vi "SPI Master and Slave with debug [FPGA].vi"() -> ()   [LabVIEW 2011]
uses:
  <vilib>/Platform/TimedLoop/XDataNode/timing_clust.ctl
  <vilib>/Platform/TimedLoop/XDataNode/nitl_modes.ctl
  <vilib>/Platform/TimedLoop/XDataNode/wakeup.ctl
  SPI Slave State.ctl
  SPI Master State.ctl
  <vilib>/rvi/interface/RandomDataEmulation/nirviRandomDataFPGAFIFO.vi
  <vilib>/rvi/interface/RandomDataEmulation/niFpgaRandomDataHandleErrors.vi
  <vilib>/Platform/TimedLoop/XDataNode/XDataNode.xnode
  <vilib>/rvi/DataTransferAndStorage/Container/XNode/niFpgaContainer.xnode
  <vilib>/rvi/interface/RandomDataEmulation/nirviRandomDataFpgaReadWriteTemplate.vi
  <vilib>/Platform/TimedLoop/XDataNode/XDNodeRunTimeDep.lvlib
panel:
  out "Slave Data Out":u32
  in  "Slave Data In":u32
  in  "Data Length":u8
  in  "HCP-1":u8
  out "Data Out":u32
  in  "Data In":u32
  in  "TX":bool
  in  "CPOL":bool
  in  "CPHA":bool
  in  "RESET":bool
  out "_SS":bool
  out "SCLK":bool
  out "MOSI":bool
  out "MISO":bool
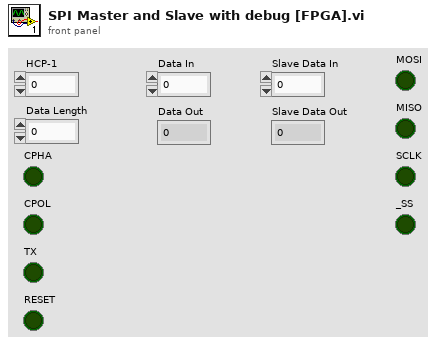
[diagram p1: front panel]
types:
  T1 = typedef "XDNodeRunTimeDep.lvlib/timing_clust.ctl" = cluster{"Expected End [f-1]":u64, "Actual End [f-1]":u64, "Finished Late? [f-1]":bool, "Expected End [i-1]":u64, "Actual End [i-1]":u64, "Finished Late? [i-1]":bool, "Expected Start [i]":u64, "Actual Start [i]":u64, "Expected Start [f]":u64, "Actual Start [f]":u64, "Source Name":string, "Structure Name":string, "Period":i64, "Deadline":i64, "Offset":i64, "Start":i64, "Priority":i32, "Timeout":i32, "Mode":T2, "Wakeup Reason":T3, "Error":errorcluster, "Source Type":string, "Secondary Source Type":string, "Global End Time":u64, "Global Start Time":u64, "Frame Duration":u64, "Iteration Duration":u64, "Assigned CPU":i32, "I/O Scan Engine Mode":u32}
  T2 = typedef "XDNodeRunTimeDep.lvlib/nitl_modes.ctl" = enum32{"No Change", "Process missed periods, maintain original phase", "Discard missed periods, maintain original phase", "Process missed periods, ignore original phase", "Discard missed periods, ignore original phase"}
  T3 = typedef "XDNodeRunTimeDep.lvlib/wakeup.ctl" = enum32{"Normal", "Aborted", "Asynchronous wakeup", "Timing source error", "Timed loop error", "Timeout"}
  T4 = typedef "SPI Slave State.ctl" = enum8{"RESET", "Wait for _SS", "Assert MISO", "Latch MOSI"}
  T5 = typedef "SPI Master State.ctl" = enum8{"RESET", "Wait for TX", "Assert MOSI", "Toggle SCLK", "Latch MISO and Toggle SCLK", "Assert MOSI and Toggle SCLK"}
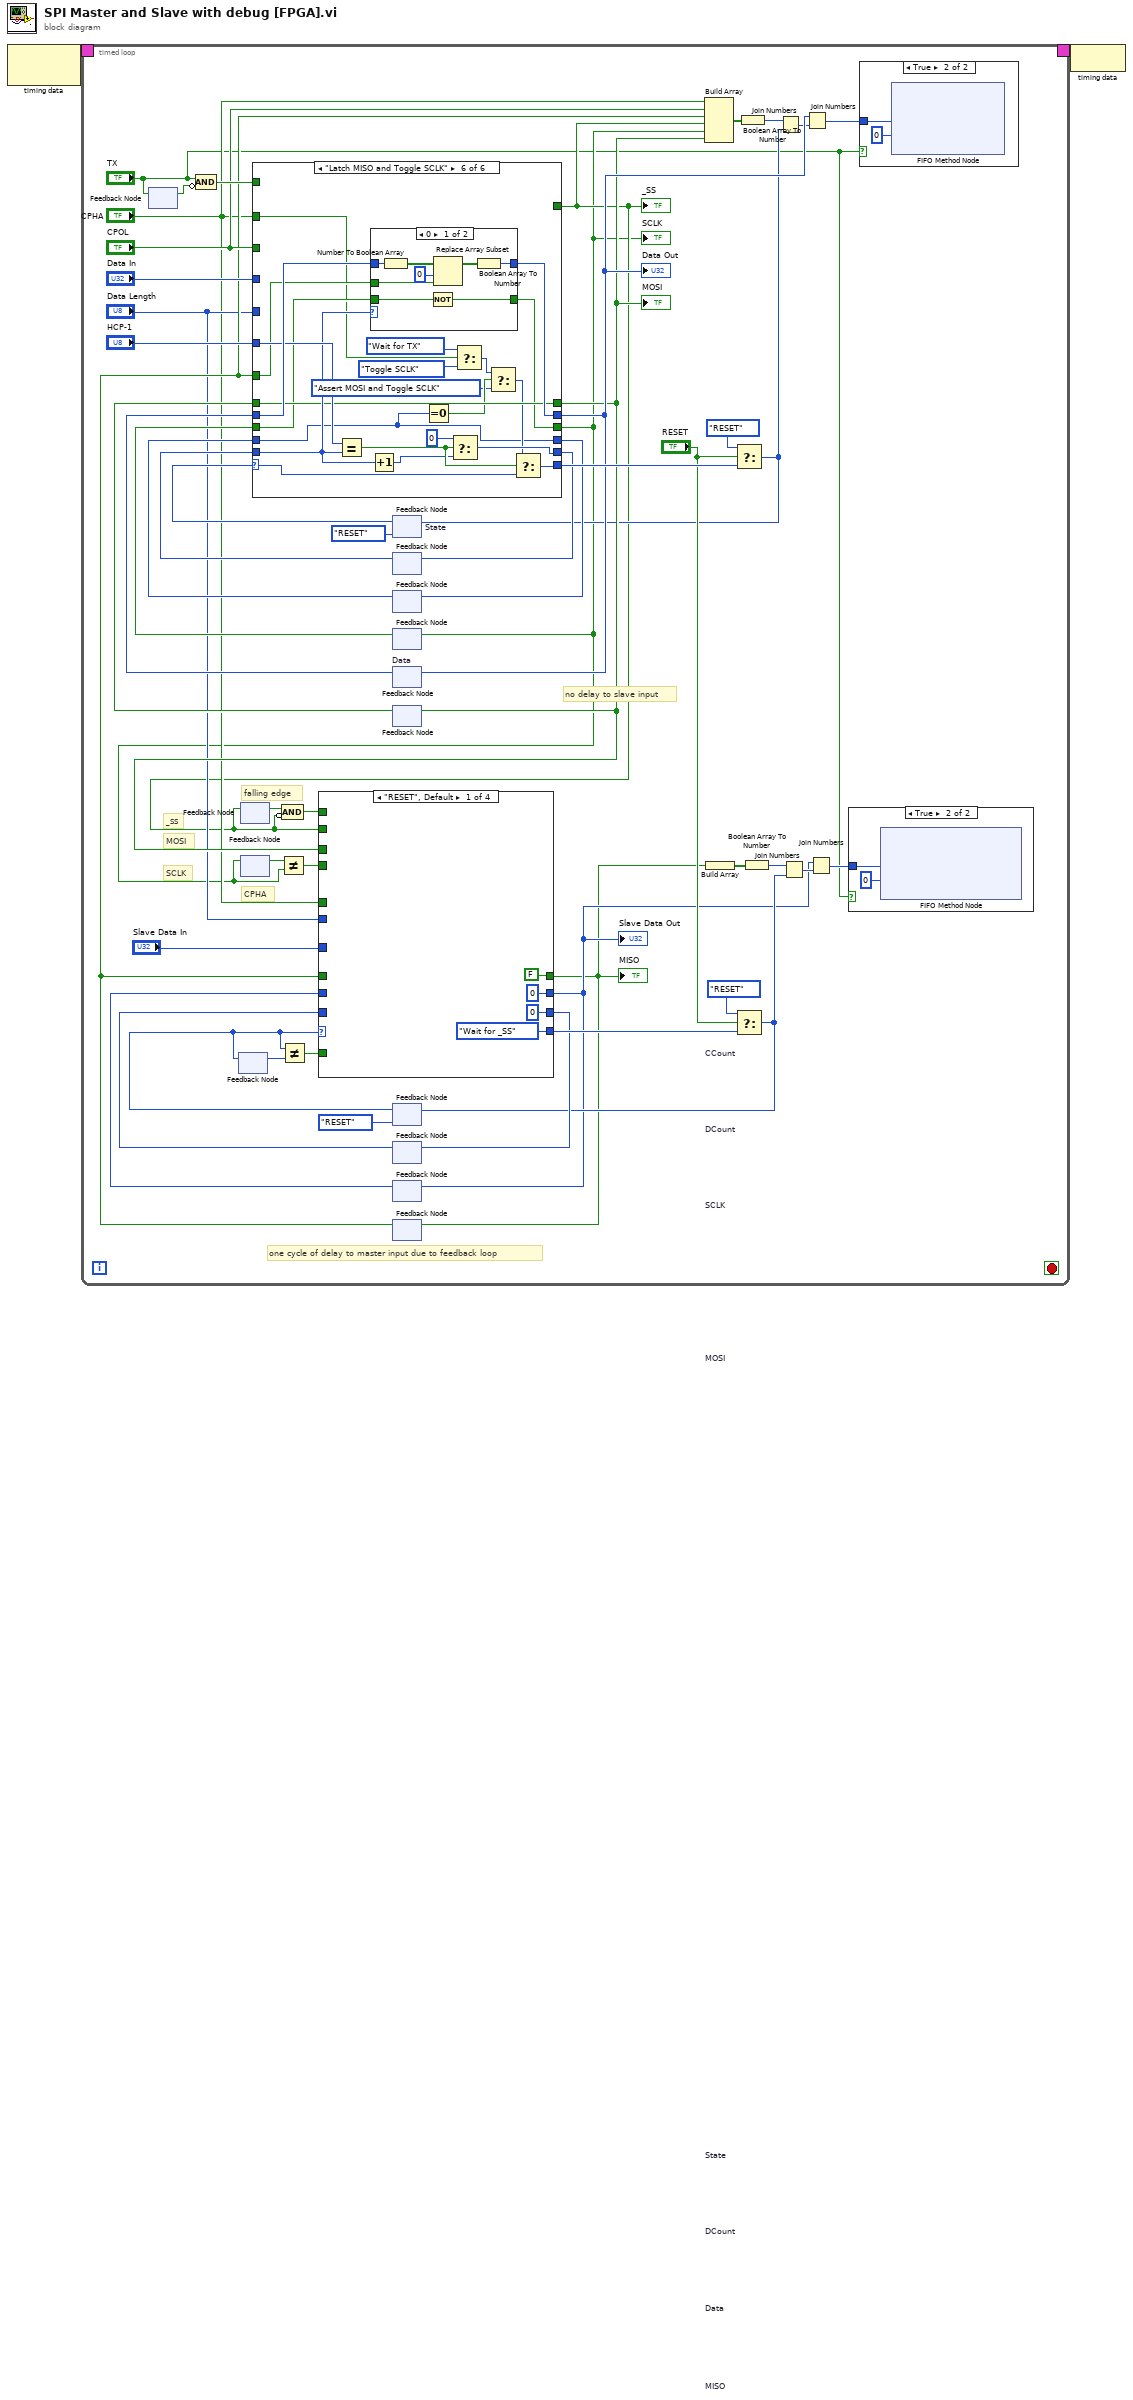
[diagram p0: block diagram]
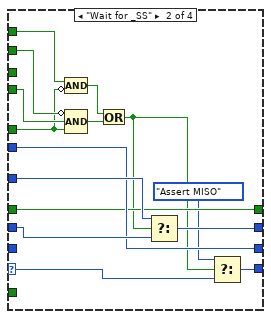
[diagram p3: hidden frame]
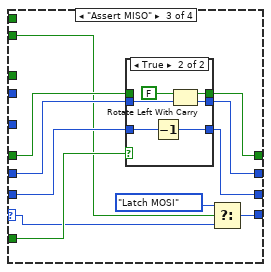
[diagram p4: hidden frame]
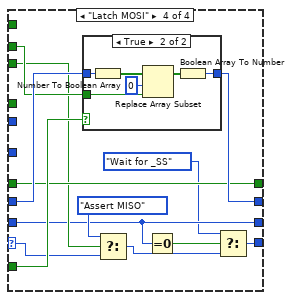
[diagram p6: hidden frame]
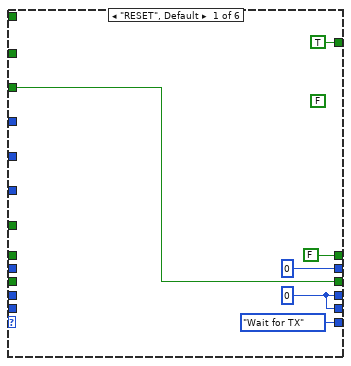
[diagram p9: hidden frame]
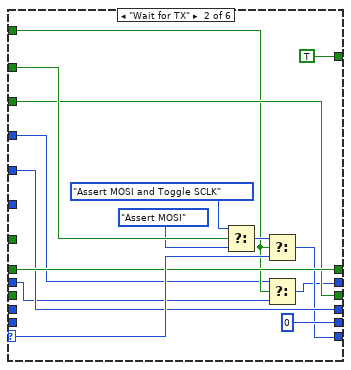
[diagram p10: hidden frame]
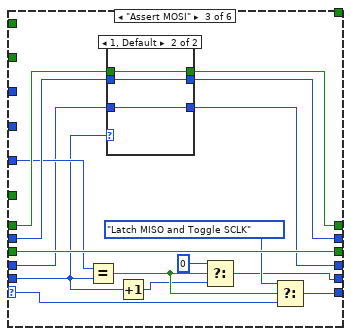
[diagram p11: hidden frame]
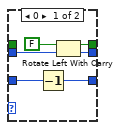
[diagram p12: hidden frame]
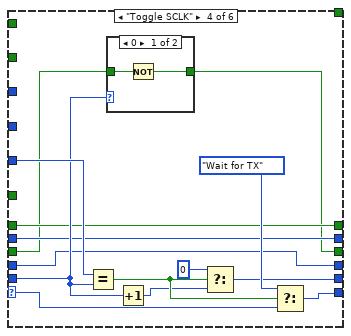
[diagram p13: hidden frame]
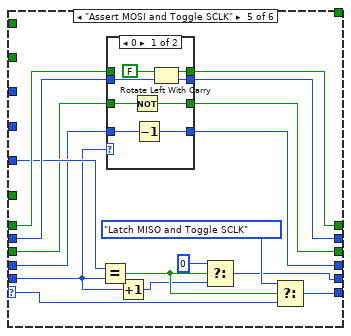
[diagram p15: hidden frame]
diagram:
  n1 = node-c288() -> (w2:T1)  [unwired: 1 in]
  n2 = timed-loop {
    timing: w2 -> [_]
    timing-out: [_] -> w1
    stop <- _ stop-if-true
    # "CPHA"
    # "falling edge"
    # "SCLK"
    # "MOSI"
    # "_SS"
    # "one cycle of delay to master input due to feedback loop"
    # "no delay to slave input"
    n3 = feedback #1() -> (w49:bool)  [unwired: 1 in]
    n4 = feedback-in #1("TX") -> ()
    n5 = Compound Arithmetic op=AND("TX", invert w49) -> (w41:bool)
    n6 = feedback #2 ("State")() -> (w13:T4)  [unwired: 1 in]
    n7 = feedback #3() -> (w19:bool)  [unwired: 1 in]
    n8 = feedback #4() -> (w16:bool)  [unwired: 1 in]
    n9 = feedback #5 "State"(SPI_Master_State."RESET") -> (w52:T5)
    n10 = feedback #6 "CCount"() -> (w46:u8)  [unwired: 1 in]
    n11 = feedback #7 "DCount"() -> (w45:u8)  [unwired: 1 in]
    n12 = feedback #8 "SCLK"() -> (w44:bool)  [unwired: 1 in]
    n13 = feedback #9 "Data"() -> (w42:u32)  [unwired: 1 in]
    n14 = feedback #10 "MOSI"() -> (w40:bool)  [unwired: 1 in]
    n15 = feedback #11 "State"(SPI_Slave_State."RESET" ("SPI Slave State")) -> (w12:T4)
    n16 = feedback-in #2(w12) -> ()
    n17 = Not Equal?(x=w12, y=w13) -> (x != y?=w11:bool)
    n18 = feedback #12 "DCount"() -> (w27:u8)  [unwired: 1 in]
    n19 = feedback #13 "Data"() -> (w24:u32)  [unwired: 1 in]
    n20 = feedback #14 "MISO"() -> (w23:bool)  [unwired: 1 in]
    n21 = case shown="\"Latch MISO and Toggle SCLK\"" w52 {
      selector: w52 -> [_ w134 w146 w174 w190 w226]
      tunnel: [SPI_Master_State."Wait for TX" w127 w147 w175 w191 w227] -> w51
      tunnel: w41 -> [_ w126 _ _ _ _]
      tunnel: [w121 u8 0 w140 w168 w184 w221] -> w48
      tunnel: [w121 w129 w138 w167 w180 w209] -> w47
      tunnel: w46 -> [_ _ w143 w171 w187 w224]
      tunnel: w45 -> [_ _ w139 w167 w181 w209]
      tunnel: [TRUE ("MOSI") TRUE ("MOSI") _ _ _ _] -> w18
      tunnel: "CPHA" -> [_ w135 _ _ _ w215]
      tunnel: [w119 w128 w149 w163 w182 w217] -> w15
      tunnel: "CPOL" -> [w119 w128 _ _ _ _]
      tunnel: w44 -> [_ _ w149 w164 w183 w218]
      tunnel: "Data In" -> [_ w125 _ _ _ _]
      tunnel: [u32 0 ("Data In") w123 w152 w166 w195 w229] -> w34
      tunnel: w42 -> [_ w124 w153 w166 w196 w230]
      tunnel: "HCP-1" -> [_ _ w148 w176 w192 w228]
      tunnel: w23 -> [_ _ _ _ _ w219]
      tunnel: "Data Length" -> [_ w129 _ _ _ _]
      tunnel: [FALSE ("msb carry out") w130 w151 w165 w194 w220] -> w31
      tunnel: w40 -> [_ w130 w150 w165 w193 w220]
      frame "RESET", Default {
        (unwired) FALSE ("msb carry out")
        w121 = u8 0
      }
      frame "Wait for TX" {
        n22 = Select(t=SPI_Master_State."Assert MOSI and Toggle SCLK", s=w135, f=SPI_Master_State."Assert MOSI" ("t")) -> (s? t:f=w131:T5)
        n23 = Select(t=w131, s=w126, f=w134) -> (s? t:f=w127:T5)
        n24 = Select(t=w125, s=w126, f=w124) -> (s? t:f=w123:u32)
      }
      frame "Assert MOSI" {
        n25 = Equal?(x=w148, y=w143) -> (x = y?=w144:bool)
        n26 = case shown="1, Default" w143 {
          tunnel: w153 -> [w158 w161]
          tunnel: [w157 w161] -> w152
          tunnel: [w156 w162] -> w151
          tunnel: w150 -> [_ w162]
          tunnel: w139 -> [w155 w160]
          tunnel: [w154 w160] -> w138
          frame 0 {
            n27 = Decrement(x=w155) -> (x-1=w154:u8)
            n28 = Rotate Left With Carry(2:w158, 3:FALSE ("carry")) -> (0:w157:u32, 1:w156:bool)
          }
          frame 1, Default {
          }
        }
        n29 = Increment(x=w143) -> (x+1=w142:u8)
        n30 = Select(t=u8 0, s=w144, f=w142) -> (s? t:f=w140:u8)
        n31 = Select(t=SPI_Master_State."Latch MISO and Toggle SCLK", s=w144, f=w146) -> (s? t:f=w147:T5)
      }
      frame "Toggle SCLK" {
        n32 = Equal?(x=w176, y=w171) -> (x = y?=w172:bool)
        n33 = case shown="0" w171 {
          tunnel: w164 -> [w178 w179]
          tunnel: [w177 w179] -> w163
          frame 0 {
            n34 = Not(x=w178) -> (.not. x?=w177:bool)
          }
          frame 1, Default {
          }
        }
        n35 = Increment(x=w171) -> (x+1=w170:u8)
        n36 = Select(t=u8 0, s=w172, f=w170) -> (s? t:f=w168:u8)
        n37 = Select(t=SPI_Master_State."Wait for TX", s=w172, f=w174) -> (s? t:f=w175:T5)
      }
      frame "Assert MOSI and Toggle SCLK" {
        n38 = Equal?(x=w192, y=w187) -> (x = y?=w188:bool)
        n39 = case shown="0" w187 {
          tunnel: w196 -> [w203 w207]
          tunnel: [w202 w207] -> w195
          tunnel: [w201 w208] -> w194
          tunnel: w193 -> [_ w208]
          tunnel: w183 -> [w200 w206]
          tunnel: [w199 w206] -> w182
          tunnel: w181 -> [w198 w205]
          tunnel: [w197 w205] -> w180
          frame 0 {
            n40 = Not(x=w200) -> (.not. x?=w199:bool)
            n41 = Decrement(x=w198) -> (x-1=w197:u8)
            n42 = Rotate Left With Carry(2:w203, 3:FALSE ("carry")) -> (0:w202:u32, 1:w201:bool)
          }
          frame 1, Default {
          }
        }
        n43 = Increment(x=w187) -> (x+1=w186:u8)
        n44 = Select(t=u8 0, s=w188, f=w186) -> (s? t:f=w184:u8)
        n45 = Select(t=SPI_Master_State."Latch MISO and Toggle SCLK", s=w188, f=w190) -> (s? t:f=w191:T5)
      }
      frame "Latch MISO and Toggle SCLK" {
        n46 = Equal?(x=w228, y=w224) -> (x = y?=w225:bool)
        n47 = Increment(x=w224) -> (x+1=w223:u8)
        n48 = case shown="0" w224 {
          tunnel: w230 -> [w238 w240]
          tunnel: [w233 w240] -> w229
          tunnel: w219 -> [w236 _]
          tunnel: w218 -> [w232 w239]
          tunnel: [w231 w239] -> w217
          frame 0 {
            n49 = Number To Boolean Array(number=w238) -> (Boolean array=w237:bool[])
            n50 = Not(x=w232) -> (.not. x?=w231:bool)
            n51 = Replace Array Subset(array=w237, new element=w236, index=0) -> (w234:bool[])
            n52 = Boolean Array To Number(Boolean array=w234) -> (number=w233:u32)
          }
          frame 1, Default {
          }
        }
        n53 = Equal To 0?(x=w209) -> (x = 0?=w216:bool)
        n54 = Select(t=u8 0, s=w225, f=w223) -> (s? t:f=w221:u8)
        n55 = Select(t=SPI_Master_State."Wait for TX", s=w215, f=SPI_Master_State."Toggle SCLK" ("t")) -> (s? t:f=w211:T5)
        n56 = Select(t=w211, s=w216, f=SPI_Master_State."Assert MOSI and Toggle SCLK" ("t")) -> (s? t:f=w213:T5)
        n57 = Select(t=w213, s=w225, f=w226) -> (s? t:f=w227:T5)
      }
    }
    "SCLK" <- w15
    "_SS" <- w18
    "MOSI" <- w31
    "Data Out" <- w34
    n58 = feedback-in #3(w18) -> ()
    n59 = feedback-in #4(w15) -> ()
    n60 = Not Equal?(x=w16, y=w15) -> (x != y?=w14:bool)
    n61 = Compound Arithmetic op=AND(w19, invert w18) -> (w17:bool)
    n62 = case shown="\"RESET\", Default" w12 {
      selector: w12 -> [_ w62 w78 w101]
      tunnel: w31 -> [_ _ _ w104]
      tunnel: [SPI_Slave_State."Wait for _SS" ("SPI Slave State") w67 w77 w98] -> w30
      tunnel: w18 -> [_ w74 _ _]
      tunnel: w27 -> [_ _ w82 w97]
      tunnel: [u8 0 w68 w81 w97] -> w26
      tunnel: [u32 0 ("Data In") w70 w80 w105] -> w4
      tunnel: w24 -> [_ w69 w84 w107]
      tunnel: w23 -> [_ w65 w83 w103]
      tunnel: [FALSE ("msb carry out") w65 w79 w103] -> w3
      tunnel: "Data Length" -> [_ w68 _ _]
      tunnel: "Slave Data In" -> [_ w71 _ _]
      tunnel: "CPHA" -> [_ w60 _ _]
      tunnel: w17 -> [_ w72 _ _]
      tunnel: w14 -> [_ w73 w76 w102]
      tunnel: w11 -> [_ _ w85 w106]
      frame "RESET", Default {
      }
      frame "Wait for _SS" {
        n63 = Compound Arithmetic op=AND(w72, invert w60) -> (w63:bool)
        n64 = Compound Arithmetic op=AND(invert w74, w73, w60) -> (w66:bool)
        n65 = Or(x=w63, y=w66) -> (x .or. y?=w61:bool)
        n66 = Select(t=w71, s=w61, f=w69) -> (s? t:f=w70:u32)
        n67 = Select(t=SPI_Slave_State."Assert MISO", s=w61, f=w62) -> (s? t:f=w67:T4)
      }
      frame "Assert MISO" {
        n68 = case shown="True" w85 {
          tunnel: w84 -> [w87 w93]
          tunnel: [w87 w92] -> w80
          tunnel: [w88 w91] -> w79
          tunnel: w83 -> [w88 _]
          tunnel: w82 -> [w86 w90]
          tunnel: [w86 w89] -> w81
          frame False {
          }
          frame True {
            n69 = Decrement(x=w90) -> (x-1=w89:u8)
            n70 = Rotate Left With Carry(2:w93, 3:FALSE ("carry")) -> (0:w92:u32, 1:w91:bool)
          }
        }
        n71 = Select(t=SPI_Slave_State."Latch MOSI", s=w76, f=w78) -> (s? t:f=w77:T4)
      }
      frame "Latch MOSI" {
        n72 = case shown="True" w106 {
          tunnel: w107 -> [w108 w114]
          tunnel: [w108 w109] -> w105
          tunnel: w104 -> [_ w112]
          frame False {
          }
          frame True {
            n73 = Number To Boolean Array(number=w114) -> (Boolean array=w113:bool[])
            n74 = Replace Array Subset(array=w113, new element=w112, index=0) -> (w110:bool[])
            n75 = Boolean Array To Number(Boolean array=w110) -> (number=w109:u32)
          }
        }
        n76 = Select(t=SPI_Slave_State."Assert MISO", s=w102, f=w101) -> (s? t:f=w99:T4)
        n77 = Equal To 0?(x=w97) -> (x = 0?=w96:bool)
        n78 = Select(t=SPI_Slave_State."Wait for _SS", s=w96, f=w99) -> (s? t:f=w98:T4)
      }
    }
    "MISO" <- w3
    "Slave Data Out" <- w4
    n79 = feedback-in #6(w48) -> ()
    n80 = feedback-in #7(w47) -> ()
    n81 = feedback-in #8(w15) -> ()
    n82 = feedback-in #9(w34) -> ()
    n83 = feedback-in #10(w31) -> ()
    n84 = feedback-in #12(w26) -> ()
    n85 = feedback-in #13(w4) -> ()
    n86 = feedback-in #14(w3) -> ()
    n87 = Build Array("CPHA", "CPOL", w23, w18, w15, w31) -> (w36:bool[])
    n88 = Build Array(w3) -> (w8:bool[])
    n89 = Select(t=SPI_Master_State."RESET", s="RESET", f=w51) -> (s? t:f=w25:T5)
    n90 = feedback-in #5(w25) -> ()
    n91 = Select(t=SPI_Slave_State."RESET", s="RESET", f=w30) -> (s? t:f=w6:T4)
    n92 = feedback-in #11(w6) -> ()
    n93 = Boolean Array To Number(Boolean array=w36) -> (number=w35:u8)
    n94 = Boolean Array To Number(Boolean array=w8) -> (number=w9:u8)
    n95 = Join Numbers(hi=w35, lo=w25) -> ((hi.lo)=w33:u16)
    n96 = Join Numbers(hi=w9, lo=w6) -> ((hi.lo)=w10:u16)
    n97 = Join Numbers(hi=w34, lo=w33) -> ((hi.lo)=w38:u64)
    n98 = Join Numbers(hi=w4, lo=w10) -> ((hi.lo)=w7:u64)
    n99 = case shown="True" "TX" {
      tunnel: w7 -> [_ w54]
      frame False {
      }
      frame True {
        n100 = xnode ("FIFO Method Node")("Element"=w54, "Timeout"=0) -> ()  [unwired: 1 in, 2 out]
      }
    }
    n101 = case shown="True" "TX" {
      tunnel: w38 -> [_ w115]
      frame False {
      }
      frame True {
        n102 = xnode ("FIFO Method Node")("Element"=w115, "Timeout"=0) -> ()  [unwired: 1 in, 2 out]
      }
    }
  }
  n103 = node-c288(w1) -> ()
